vi "Main.vi"() -> ()   [LabVIEW 2018]
doc: "The myRIO Project template acquires acceleration data from the onboard accelerometer and displays the changes of acceleration values in a waveform chart."
uses:
  <vilib>/Platform/TimedLoop/XDataNode/timing_clust.ctl
  <vilib>/Platform/TimedLoop/XDataNode/nitl_modes.ctl
  <vilib>/Platform/TimedLoop/XDataNode/wakeup.ctl
  <vilib>/myRIO/Instrument Drivers/Onboard IO/DIO/typedefs/DIO Reference.ctl
  <vilib>/myRIO/Common/Instrument Driver Framework/Utilities/typedefs/myRIO Generic Hardware Reference.ctl
  <vilib>/myRIO/Common/Instrument Driver Framework/Utilities/typedefs/Hardware Version Enum.ctl
  <vilib>/myRIO/Common/Instrument Driver Framework/Utilities/typedefs/myRIO v1.0 Reference.ctl
  <vilib>/myRIO/Common/Instrument Driver Framework/Utilities/typedefs/Generic FPGA Reference.ctl
  <vilib>/myRIO/Common/Instrument Driver Framework/myRIO v1.0/DIO/typedefs/DIO Channels List.ctl
  <vilib>/myRIO/Common/Instrument Driver Framework/myRIO v1.0/DIO/typedefs/DIO Channels Enum.ctl
  <vilib>/userdefined/High Color/nirio_resource_hc.ctl
  <vilib>/myRIO/Instrument Drivers/Onboard IO/AI/typedefs/AI Reference.ctl
  <vilib>/myRIO/Common/Instrument Driver Framework/myRIO v1.0/AI/typedefs/AI Channels List.ctl
  <vilib>/myRIO/Common/Instrument Driver Framework/myRIO v1.0/AI/typedefs/AI Channels Enum.ctl
  <vilib>/myRIO/Common/Instrument Driver Framework/Utilities/typedefs/Analog Scaling Constants List.ctl
  <vilib>/myRIO/Common/Instrument Driver Framework/Utilities/typedefs/Analog Scaling Constants.ctl
  <vilib>/myRIO/Instrument Drivers/Onboard IO/AO/typedefs/AO Reference.ctl
  <vilib>/myRIO/Common/Instrument Driver Framework/myRIO v1.0/AO/typedefs/AO Channels List.ctl
  <vilib>/myRIO/Common/Instrument Driver Framework/myRIO v1.0/AO/typedefs/AO Channels Enum.ctl
  <vilib>/myRIO/Common/Instrument Driver Framework/Utilities/vis/Is FPGA Ref Available.vi
  <vilib>/myRIO/Common/Instrument Driver Framework/myRIO v1.0/AI/vis/myRIO v1.1 Open AI.vi
  <vilib>/myRIO/Instrument Drivers/Onboard IO/AI/vis/Read.vi
  <vilib>/myRIO/Common/Instrument Driver Framework/myRIO v1.0/AO/vis/myRIO v1.1 Open AO.vi
  <vilib>/myRIO/Instrument Drivers/Onboard IO/AO/vis/Write.vi
  <vilib>/myRIO/Common/Instrument Driver Framework/myRIO v1.0/DIO/vis/myRIO v1.1 Open DIO.vi
  <vilib>/myRIO/Instrument Drivers/Onboard IO/DIO/vis/Write.vi
  <vilib>/myRIO/Instrument Drivers/Onboard IO/DIO/vis/Read.vi
  <vilib>/myRIO/Common/Instrument Driver Framework/Utilities/vis/Validate Channels.vi
  <vilib>/myRIO/Common/Instrument Driver Framework/myRIO v1.0/AI/vis/myRIO v1.0 Reserve AI.vi
  <vilib>/myRIO/Common/Instrument Driver Framework/myRIO v1.0/AO/vis/myRIO v1.0 Reserve AO.vi
  <vilib>/myRIO/Common/Instrument Driver Framework/myRIO v1.0/DIO/vis/myRIO v1.0 Reserve DIO.vi
  <vilib>/myRIO/Common/Instrument Driver Framework/myRIO v1.0/AI/vis/myRIO v1.0 Build MUX Configuration AI.vi
  <vilib>/myRIO/Common/Instrument Driver Framework/myRIO v1.0/Resource Manager/vis/myRIO v1.0 Reserve Channel List.vi
  <vilib>/myRIO/Common/Instrument Driver Framework/myRIO v1.0/AO/vis/myRIO v1.0 Build MUX Configuration AO.vi
  <vilib>/myRIO/Common/Instrument Driver Framework/myRIO v1.0/DIO/vis/myRIO v1.0 Build MUX Configuration DIO.vi
  <vilib>/myRIO/Common/Instrument Driver Framework/myRIO v1.0/Resource Manager/vis/myRIO v1.0 Reserve Channel.vi
  <vilib>/myRIO/Common/Instrument Driver Framework/myRIO v1.0/Resource Manager/vis/myRIO v1.0 Unreserve Channel.vi
  <vilib>/myRIO/Common/Instrument Driver Framework/myRIO v1.0/Resource Manager/vis/myRIO v1.0 Create Configuration List.vi
  <vilib>/myRIO/Common/Instrument Driver Framework/myRIO v1.0/Resource Manager/vis/myRIO v1.0 Build Mutex Name.vi
  <vilib>/functionblocks/Counter/Pulse Timer/Pulse Timer.vi
  <vilib>/Utility/VariantDataType/GetNumericInfo.vi
  <vilib>/Utility/error.llb/Error Cluster From Error Code.vi
  <vilib>/myRIO/Common/Instrument Driver Framework/myRIO v1.0/myRIO v1.1 Open.vi
  <vilib>/myRIO/Common/Instrument Driver Framework/myRIO v1.0/AI/vis/myRIO v1.0 Get Scaling Constants AI.vi
  <vilib>/myRIO/Common/Instrument Driver Framework/Utilities/vis/IO Manager.vi
  <vilib>/myRIO/Common/Instrument Driver Framework/Utilities/vis/Configuration Manager.vi
  <vilib>/myRIO/Common/Instrument Driver Framework/myRIO v1.0/myRIO v1.0 Close.vi
  <vilib>/myRIO/Common/Instrument Driver Framework/myRIO v1.0/AI/vis/myRIO v1.0 Read AI.vi
  <vilib>/myRIO/Common/Instrument Driver Framework/myRIO v1.0/Resource Manager/vis/myRIO v1.0 Configure IO.vi
  <vilib>/myRIO/Common/Instrument Driver Framework/myRIO v1.0/DIO/vis/myRIO v1.0 Write DIO.vi
  <vilib>/myRIO/Common/Instrument Driver Framework/myRIO v1.0/DIO/vis/myRIO v1.0 Read DIO.vi
  <vilib>/functionblocks/Bistables/SR Bistable/SR Bistable.vi
  <vilib>/myRIO/Common/Instrument Driver Framework/myRIO v1.0/AO/vis/myRIO v1.0 Get Scaling Constants AO.vi
  <vilib>/myRIO/Common/Instrument Driver Framework/myRIO v1.0/AO/vis/myRIO v1.0 Write AO.vi
  <vilib>/Utility/file.llb/Write Delimited Spreadsheet (string).vi
  <vilib>/Platform/TimedLoop/XDataNode/XDataNode.xnode
  <vilib>/functionblocks/FB Core/FB Core.xnode
  <vilib>/myRIO/Express VI/Onboard IO/AI/AI Express VI.xnode
  <vilib>/myRIO/Instrument Drivers/Onboard IO/AI/vis/myRIO AI Open.xnode
  <vilib>/myRIO/Express VI/Onboard IO/DO/DO Express VI.xnode
  <vilib>/myRIO/Instrument Drivers/Onboard IO/DIO/vis/myRIO DIO Open.xnode
  <vilib>/myRIO/Express VI/Onboard IO/DI/DI Express VI.xnode
  <vilib>/myRIO/Express VI/Onboard IO/AO/AO Express VI.xnode
  <vilib>/myRIO/Instrument Drivers/Onboard IO/AO/vis/myRIO AO Open.xnode
  <vilib>/myRIO/Express VI/Onboard Devices/LED/LED Express VI.xnode
  <vilib>/myRIO/Instrument Drivers/Onboard IO/DIO/DIO.lvlib
  <vilib>/myRIO/Instrument Drivers/Onboard IO/AI/AI.lvlib
  <vilib>/myRIO/Instrument Drivers/Onboard IO/AO/AO.lvlib
  <vilib>/functionblocks/NI_FunctionBlock Libraries.lvlib
  <vilib>/Platform/TimedLoop/XDataNode/XDNodeRunTimeDep.lvlib
panel:
  out "AOUT":dbl
  out "AIN":dbl
  in  "Pump Test":bool
  out "APPS fault":bool
  out "APPS Output (V)":dbl
  out "APPS output %":dbl
  out "Accelaration":dbl(knob) scale=0.0..100.0
  out "APPS pedal travel %":dbl
  out "APPS2 (V) Input (B/AI1 (Pin 5)) 2":dbl
  out "APPS1":dbl(knob) scale=0.0..100.0
  out "APPS2":dbl(knob) scale=0.0..100.0
  out "APPS2 % 2":dbl
  out "APPS1 (V) Input (B/AI1 (Pin 5)) 2":dbl
  out "APPS1 % 2":dbl
  out "Pump out":bool
  out "RTD Status LED":bool
  out "RFE Indicator":bool
  out "AIR + Boolean":bool
  out "AIR +(A9)":dbl
  out "RTD Button":bool
  out "RTD Brake":bool
  out "EN Indicator":bool
  out "RTD Buzzer":bool
  in  "Buzzer test":bool
  in  "RTD Brake Test":bool
  in  "RFE  Test":bool
  in  "EN Test":bool
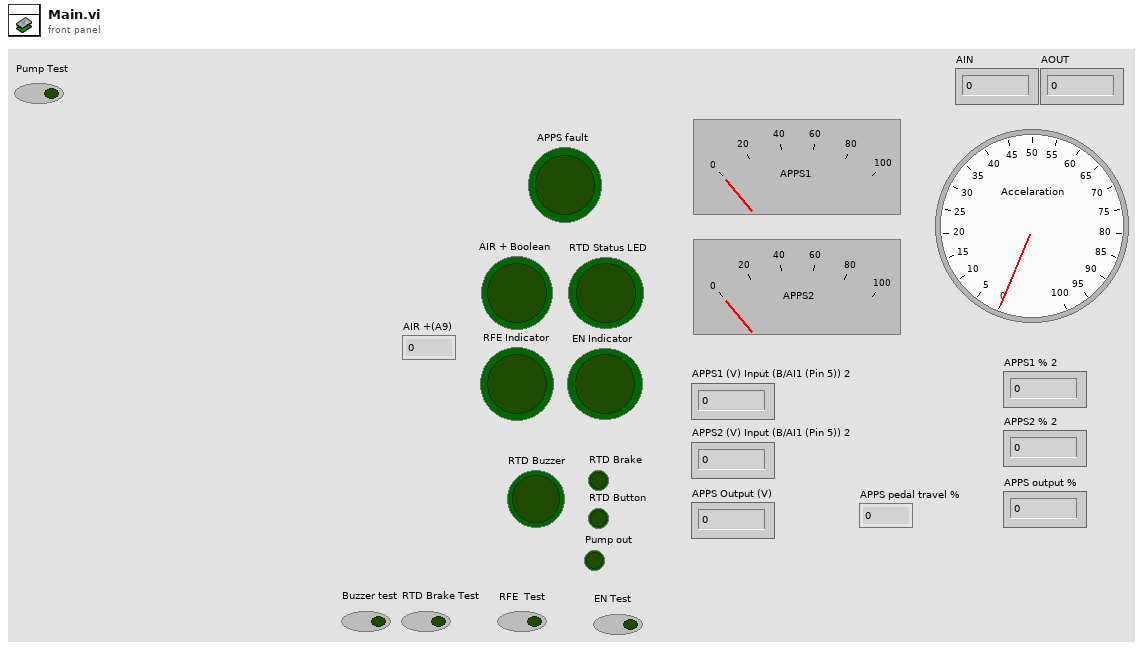
[diagram p1: front panel]
types:
  T1 = typedef "XDNodeRunTimeDep.lvlib/timing_clust.ctl" = cluster{"Expected End [f-1]":u64, "Actual End [f-1]":u64, "Finished Late? [f-1]":bool, "Expected End [i-1]":u64, "Actual End [i-1]":u64, "Finished Late? [i-1]":bool, "Expected Start [i]":u64, "Actual Start [i]":u64, "Expected Start [f]":u64, "Actual Start [f]":u64, "Source Name":string, "Structure Name":string, "Period":i64, "Deadline":i64, "Offset":i64, "Start":i64, "Priority":i32, "Timeout":i32, "Mode":T2, "Wakeup Reason":T3, "Error":errorcluster, "Source Type":string, "Secondary Source Type":string, "Global End Time":u64, "Global Start Time":u64, "Frame Duration":u64, "Iteration Duration":u64, "Assigned CPU":i32, "I/O Scan Engine Mode":u32}
  T2 = typedef "XDNodeRunTimeDep.lvlib/nitl_modes.ctl" = enum32{"No Change", "Process missed periods, maintain original phase", "Discard missed periods, maintain original phase", "Process missed periods, ignore original phase", "Discard missed periods, ignore original phase"}
  T3 = typedef "XDNodeRunTimeDep.lvlib/wakeup.ctl" = enum32{"Normal", "Aborted", "Asynchronous wakeup", "Timing source error", "Timed loop error", "Timeout"}
  T4 = typedef "AO.lvlib/AO Reference.ctl" = cluster{"myRIO Reference":T5, "AO Channel List":T9, "AO Scaling Constant List":T11}
  T5 = typedef "myRIO Generic Hardware Reference.ctl" = cluster{"myRIO Model":T6, "myRIO Hardware Reference":T7}
  T6 = typedef "Hardware Version Enum.ctl" = enum16{"Unknown", "myRIO-1900", "myRIO-1950", "roboRIO", "NI ELVIS RIO CM", "ELVIS III"}
  T7 = typedef "myRIO v1.0 Reference.ctl" = cluster{"Generic FPGA Reference":T8, "Allow multiple opens":bool}
  T8 = typedef "Generic FPGA Reference.ctl" = refnum<k20>
  T9 = typedef "AO Channels List.ctl" = T10[]
  T10 = typedef "AO Channels Enum.ctl" = enum16{"Not Connected", "AudioOut/Left", "AudioOut/Right", "C/AO0", "C/AO1", "A/AO0", "A/AO1", "B/AO0", "B/AO1"}
  T11 = typedef "Analog Scaling Constants List.ctl" = T12[]
  T12 = typedef "Analog Scaling Constants.ctl" = cluster{"LSB Weight (Volts)":dbl, "Offset (Volts)":dbl, "Signed?":bool}
  T13 = typedef "nirio_resource_hc.ctl" = tag
  T14 = typedef "AI.lvlib/AI Reference.ctl" = cluster{"myRIO Reference":T5, "AI Channels List":T15, "AI Scaling Constants List":T11}
  T15 = typedef "AI Channels List.ctl" = T16[]
  T16 = typedef "AI Channels Enum.ctl" = enum16{"Not Connected", "AudioIn/Left", "AudioIn/Right", "C/AI0", "C/AI1", "A/AI0", "A/AI1", "A/AI2", "A/AI3", "A/AI4", "A/AI5", "A/AI6", "A/AI7", "B/AI0", "B/AI1", "B/AI2", "B/AI3", "B/AI4", "B/AI5", "B/AI6", "B/AI7", "AI/AI0", "AI/AI1", "AI/AI2", "AI/AI3", "A/AI0 (DIFF)", "A/AI1 (DIFF)", "A/AI2 (DIFF)", "A/AI3 (DIFF)", "B/AI0 (DIFF)", "B/AI1 (DIFF)", "B/AI2 (DIFF)", "B/AI3 (DIFF)"}
  T17 = typedef "DIO.lvlib/DIO Reference.ctl" = cluster{"myRIO Reference":T5, "DIO Channels List":T18}
  T18 = typedef "DIO Channels List.ctl" = T19[]
  T19 = typedef "DIO Channels Enum.ctl" = enum16{"Not Connected", "C/DIO0", "C/DIO1", "C/DIO2", "C/DIO3", "C/DIO4", "C/DIO5", "C/DIO6", "C/DIO7", "A/DIO0", "A/DIO1", "A/DIO2", "A/DIO3", "A/DIO4", "A/DIO5", "A/DIO6", "A/DIO7", "A/DIO8", "A/DIO9", "A/DIO10", "A/DIO11", "A/DIO12", "A/DIO13", "A/DIO14", "A/DIO15", "A/DIO16", "A/DIO17", "A/DIO18", "A/DIO19", "B/DIO0", "B/DIO1", "B/DIO2", "B/DIO3", "B/DIO4", "B/DIO5", "B/DIO6", "B/DIO7", "B/DIO8", "B/DIO9", "B/DIO10", "B/DIO11", "B/DIO12", "B/DIO13", "B/DIO14", "B/DIO15", "B/DIO16", "B/DIO17", "B/DIO18", "B/DIO19", "LED0", "LED1", "LED2", "LED3", "Button0", "DIO/DIO0", "DIO/DIO1", "DIO/DIO2", "DIO/DIO3", "DIO/DIO4", "DIO/DIO5", "DIO/DIO6", "DIO/DIO7", "DIO/DIO8", "DIO/DIO9", "SPI/CS0", "SPI/CS1", "SPI/CS2", "SPI/CS3", "LED RADIO (Green)", "LED RADIO (Red)", "LED COMM (Green)", "LED COMM (Red)", "LED MODE (Green)", "LED MODE (Red)"}
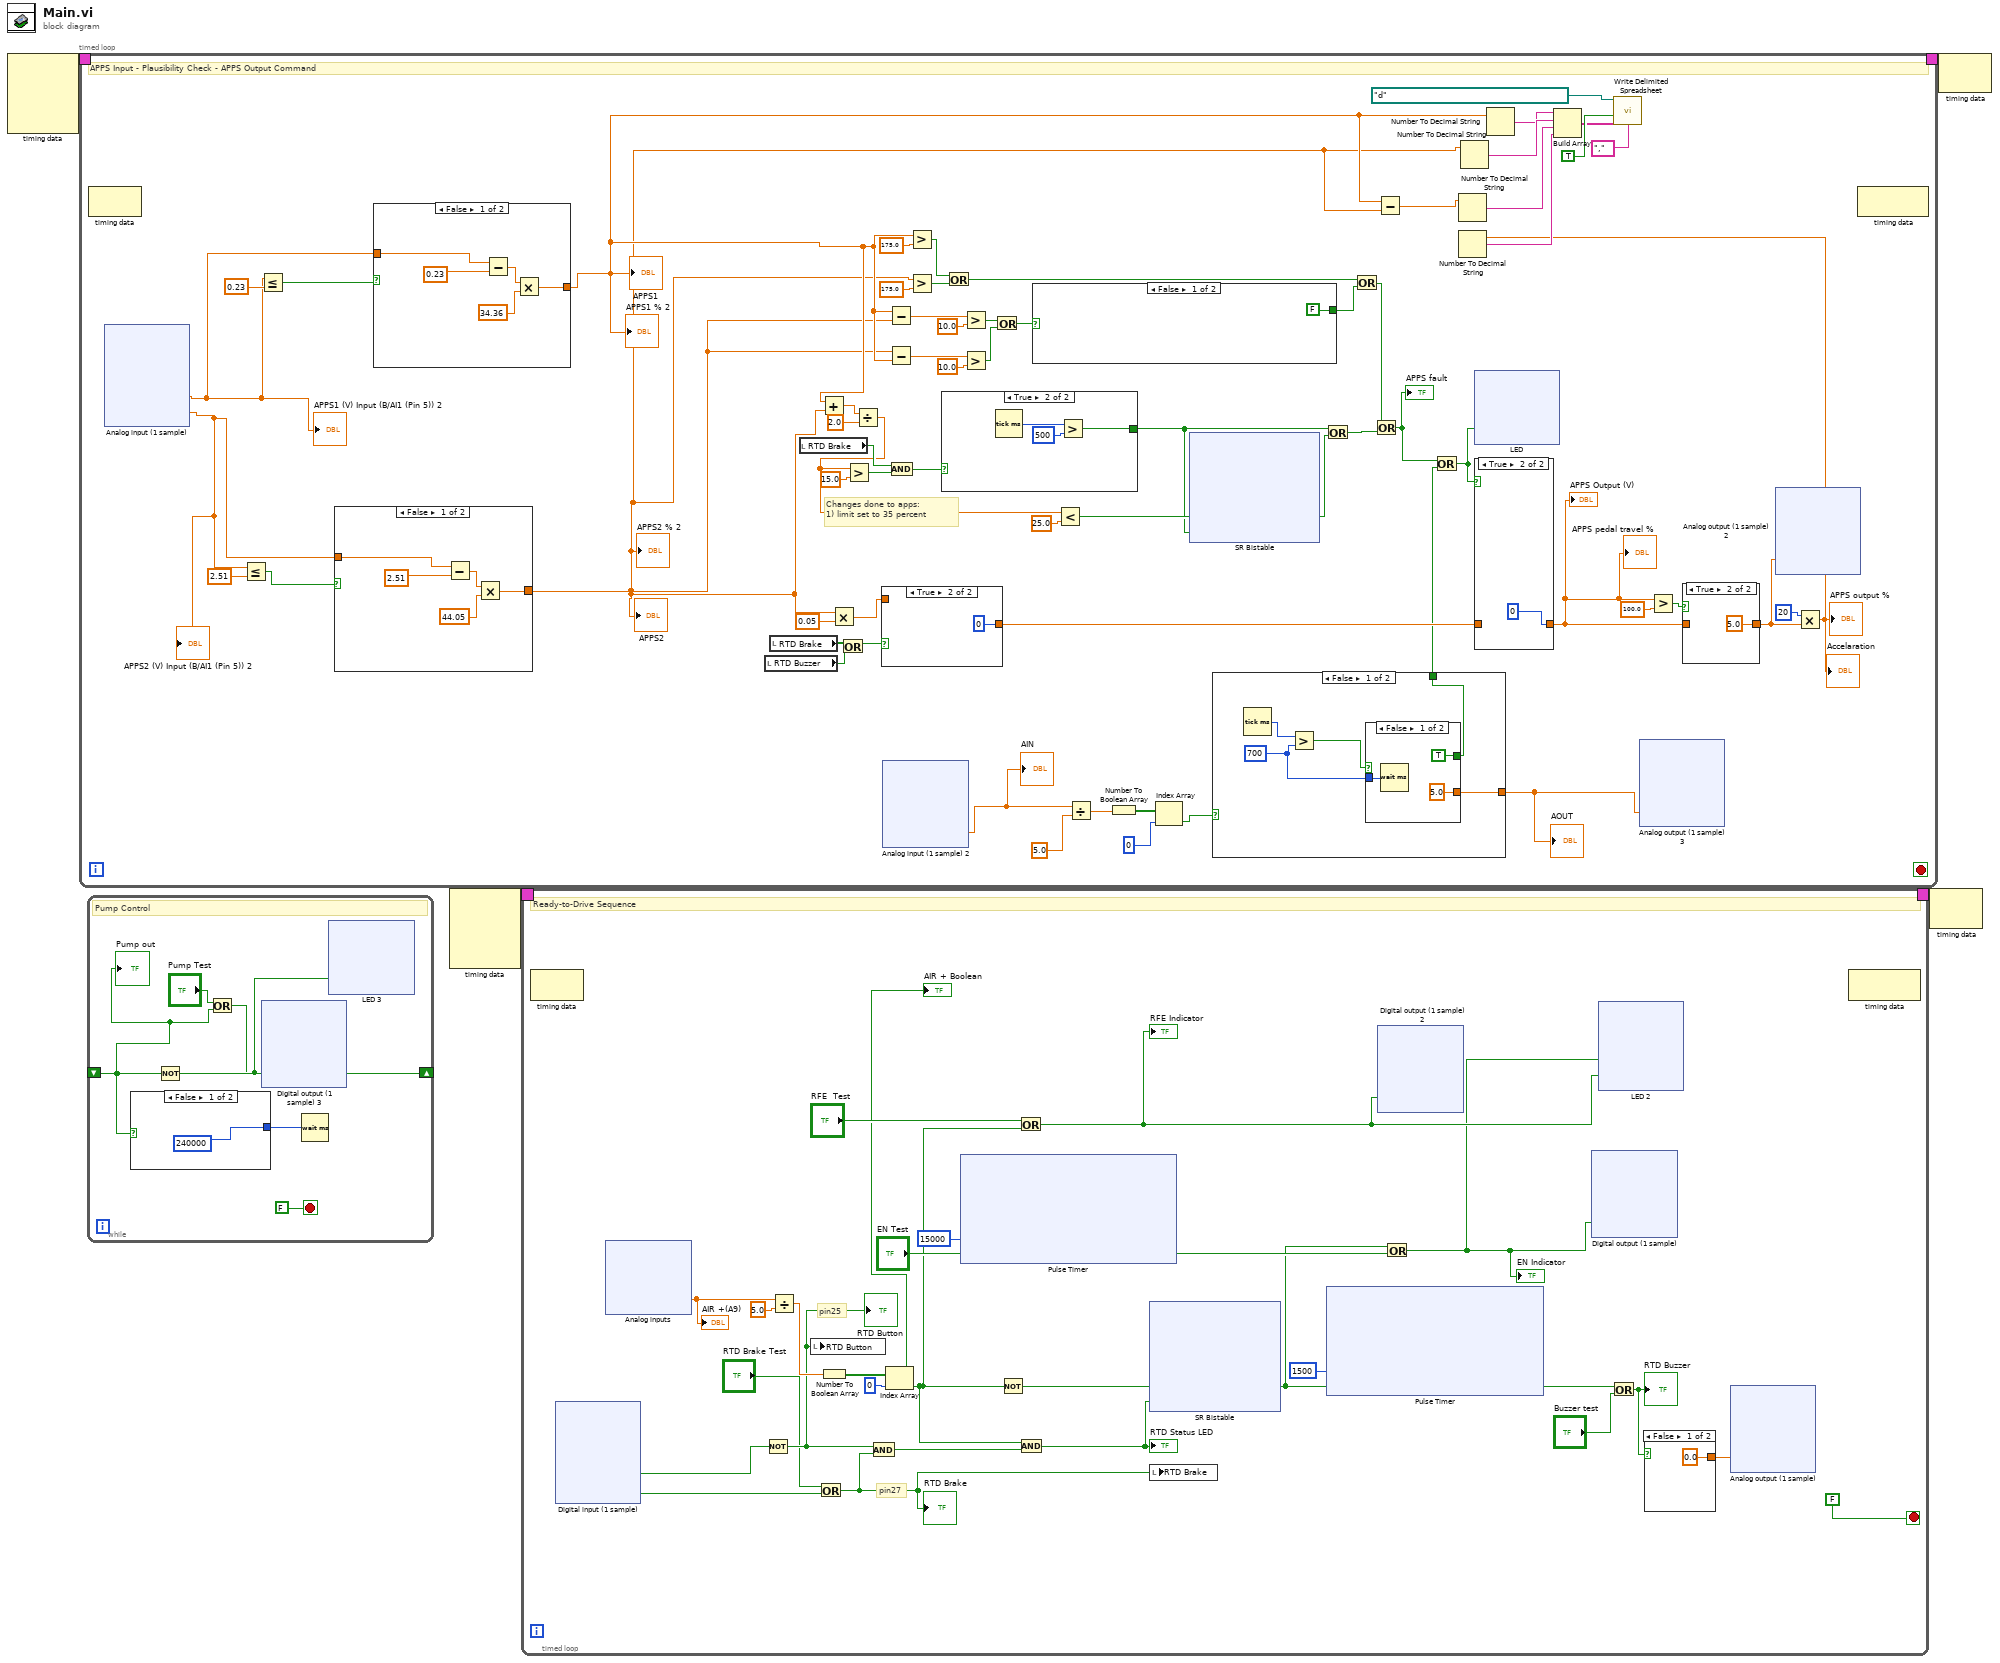
[diagram p0: block diagram]
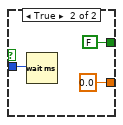
[diagram p2: hidden frame]
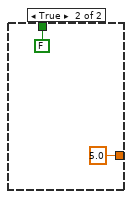
[diagram p3: hidden frame]
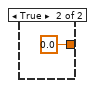
[diagram p4: hidden frame]
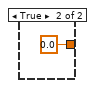
[diagram p5: hidden frame]
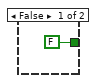
[diagram p6: hidden frame]
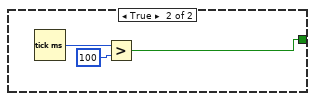
[diagram p7: hidden frame]
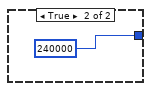
[diagram p11: hidden frame]
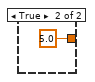
[diagram p12: hidden frame]
diagram:
  n1 = node-c288() -> (w2:T1)  [unwired: 4 in]
  n2 = timed-loop {
    timing: w2 -> [_]
    timing-out: [_] -> w1
    stop <- _ stop-if-true
    # "Changes done to apps:\n1) limit set to 35 percent"
    # "APPS Input - Plausibility Check - APPS Output Command"
    n3 = node-c288() -> ()  [unwired: 1 in, 1 out]
    n4 = xnode "Analog input (1 sample)"() -> ("APPS 1 Input (A/AI2 (Pin 7))"=w16:dbl, "APPS 2 Input (A/AI1 (Pin 5))"=w15:dbl)  [unwired: 1 in, 1 out]
    "APPS2 (V) Input (B/AI1 (Pin 5)) 2" <- w15
    "APPS1 (V) Input (B/AI1 (Pin 5)) 2" <- w16
    n5 = Less Or Equal?(x=w15, y=2.51) -> (x <= y?=w35:bool)
    n6 = Less Or Equal?(x=w16, y=0.23) -> (x <= y?=w33:bool)
    n7 = case shown="False" w35 {
      tunnel: w15 -> [w163 _]
      tunnel: [w162 0.0] -> w21
      frame False {
        n8 = Subtract(x=w163, y=2.51) -> (x-y=w165:dbl)
        n9 = Multiply(x=w165, y=44.05) -> (x*y=w162:dbl)
      }
      frame True {
      }
    }
    "APPS2" <- w21
    "APPS2 % 2" <- w21
    n10 = case shown="False" w33 {
      tunnel: w16 -> [w157 _]
      tunnel: [w156 0.0] -> w22
      frame False {
        n11 = Subtract(x=w157, y=0.23) -> (x-y=w159:dbl)
        n12 = Multiply(x=w159, y=34.36) -> (x*y=w156:dbl)
      }
      frame True {
      }
    }
    "APPS1" <- w22
    "APPS1 % 2" <- w22
    n13 = local read "RTD Buzzer"() -> (w38:bool)
    n14 = local read "RTD Brake"() -> (w32:bool)
    n15 = local read "RTD Brake"() -> (w46:bool)
    n16 = Add(x=w22, y=w21) -> (x+y=w41:dbl)
    n17 = Multiply(x=w21, y=0.05) -> (x*y=w29:dbl)
    n18 = Or(x=w32, y=w38) -> ()  [unwired: 1 out]
    n19 = Divide(x=w41, y=2.0) -> (x/y=w39:dbl)
    n20 = Greater?(x=w39, y=15.0) -> (0:w56:bool)
    n21 = case shown="True" w32 {
      tunnel: [w258 0] -> w53
      tunnel: w29 -> [w258 _]
      frame False {
      }
      frame True {
      }
    }
    n22 = xnode "Analog input (1 sample) 2"() -> ("AI (A/AI0 (Pin 3))"=w14:dbl)  [unwired: 1 in, 1 out]
    "AIN" <- w14
    n23 = Subtract(x=w22, y=w21) -> (x-y=w66:dbl)
    n24 = Subtract(x=w21, y=w22) -> (x-y=w58:dbl)
    n25 = And(x=w46, y=w56) -> (x .and. y?=w43:bool)
    n26 = Greater?(x=w22, y=175.0) -> (0:w63:bool)
    n27 = Greater?(x=w21, y=175.0) -> (0:w62:bool)
    n28 = case shown="True" w43 {
      tunnel: [FALSE w209] -> w42
      frame False {
      }
      frame True {
        n29 = Tick Count (ms)() -> (millisecond timer value=w211:u32)
        n30 = Greater?(x=w211, y=u32 500) -> (0:w209:bool)
      }
    }
    n31 = Or(x=w63, y=w62) -> (x .or. y?=w61:bool)
    n32 = Greater?(x=w66, y=10.0) -> (0:w67:bool)
    n33 = Greater?(x=w58, y=10.0) -> (0:w59:bool)
    n34 = Or(x=w67, y=w59) -> (x .or. y?=w50:bool)
    n35 = case shown="False" w50 {
      tunnel: [FALSE w255] -> w49
      frame False {
      }
      frame True {
        n36 = Tick Count (ms)() -> (millisecond timer value=w257:u32)
        n37 = Greater?(x=w257, y=u32 100) -> (0:w255:bool)
      }
    }
    n38 = Less?(x=w39, y=25.0) -> (x < y?=w47:bool)
    n39 = Divide(x=w14, y=5.0) -> (x/y=w12:dbl)
    n40 = Number To Boolean Array(number=w12) -> (Boolean array=w11:bool[])
    n41 = Index Array(array=w11, index=0) -> (element=w9:bool)
    n42 = xnode "SR Bistable"("reset"=w47, "set"=w42) -> ("output"=w48:bool)  [unwired: 1 in, 1 out]
    n43 = case shown="False" w9 {
      tunnel: [w108 5.0] -> w5
      tunnel: [w107 FALSE] -> w8
      frame False {
        w106 = u32 700 ("y")
        n44 = Tick Count (ms)() -> (millisecond timer value=w109:u32)
        n45 = Greater?(x=w109, y=w106) -> (0:w110:bool)
        n46 = case shown="False" w110 {
          tunnel: [5.0 0.0] -> w108
          tunnel: [TRUE FALSE] -> w107
          tunnel: w106 -> [w111 w114]
          frame False {
            n47 = Wait (ms)(milliseconds to wait=w111) -> ()  [unwired: 1 out]
          }
          frame True {
            n48 = Wait (ms)(milliseconds to wait=w114) -> ()  [unwired: 1 out]
          }
        }
      }
      frame True {
      }
    }
    "AOUT" <- w5
    n49 = Or(x=w42, y=w48) -> (x .or. y?=w44:bool)
    n50 = Or(x=w61, y=w49) -> (x .or. y?=w45:bool)
    n51 = Or(x=w45, y=w44) -> (x .or. y?=w7:bool)
    "APPS fault" <- w7
    n52 = Subtract(x=w22, y=w21) -> (x-y=w20:dbl)
    n53 = Or(x=w7, y=w8) -> (x .or. y?=w6:bool)
    n54 = Number To Decimal String(number=w20) -> (decimal integer string=w23:string)  [unwired: 1 in]
    n55 = Number To Decimal String(number=w21) -> (decimal integer string=w28:string)  [unwired: 1 in]
    n56 = xnode "LED"("LED0"=w6) -> ()  [unwired: 1 in, 1 out]
    n57 = case shown="True" w6 {
      tunnel: w53 -> [w262 _]
      tunnel: [w262 0] -> w31
      frame False {
      }
      frame True {
      }
    }
    "APPS Output (V)" <- w31
    "APPS pedal travel %" <- w31
    n58 = Number To Decimal String(number=w22) -> (decimal integer string=w27:string)  [unwired: 1 in]
    n59 = xnode "Analog output (1 sample) 3"("A/AO0 (Pin 2)"=w5) -> ()  [unwired: 1 in, 1 out]
    n60 = Greater?(x=w31, y=100.0) -> (0:w54:bool)
    n61 = case shown="True" w54 {
      tunnel: [w260 5.0 ("APPS output %")] -> w37
      tunnel: w31 -> [w260 _]
      frame False {
      }
      frame True {
      }
    }
    n62 = xnode "Analog output (1 sample) 2"("APPS Output (B/AO0 (Pin 2))"=w37) -> ()  [unwired: 1 in, 1 out]
    n63 = Multiply(x=20, y=w37) -> (x*y=w18:dbl)
    "APPS output %" <- w18
    "Accelaration" <- w18
    n64 = Number To Decimal String(number=w18) -> (decimal integer string=w19:string)  [unwired: 1 in]
    n65 = Build Array(w27, w28, w23, w19) -> (w17:string[])
    n66 = call-poly <vilib>:"Write Delimited Spreadsheet.vi"("file path (dialog if empty)"=path "d:/", "1D data"=w17, "append to file? (new file:F)"=TRUE, "delimiter (\\t)"="," ("delimiter (\\t)")) -> ()  [unwired: 10 in, 2 out]
    n67 = node-c288() -> ()  [unwired: 1 in, 1 out]
  }
  n68 = while {
    shift-right: [w341] -> _
    shift-left: _ -> [w337]
    stop <- FALSE stop-if-true
    # "Pump Control"
    n69 = case shown="False" w337 {
      tunnel: [240000 240000] -> w340
      frame False {
      }
      frame True {
      }
    }
    n70 = Not(x=w337) -> (.not. x?=w341:bool)
    n71 = Or(x="Pump Test", y=w337) -> (x .or. y?=w336:bool)
    n72 = xnode "Digital output (1 sample) 3"("Pump out (B/DIO7 (Pin 25))"=w336) -> ()  [unwired: 1 in, 1 out]
    n73 = Wait (ms)(milliseconds to wait=w340) -> ()  [unwired: 1 out]
    n74 = xnode "LED 3"("PUMP"=w336) -> ()  [unwired: 1 in, 1 out]
    "Pump out" <- w337
  }
  n75 = node-c288() -> (w4:T1)  [unwired: 4 in]
  n76 = timed-loop {
    timing: w4 -> [_]
    timing-out: [_] -> w3
    stop <- FALSE stop-if-true
    # "pin27"
    # "pin25"
    # "Ready-to-Drive Sequence"
    n77 = node-c288() -> ()  [unwired: 1 in, 1 out]
    n78 = xnode "Digital input (1 sample)"() -> ("RTD Button (B/DIO2 (Pin 15))"=w435:bool, "RTD Brake (B/DIO3 (Pin 17))"=w416:bool)  [unwired: 1 in, 1 out]
    n79 = xnode "Analog inputs"() -> ("AIR + (A/AI3 (Pin 9))"=w419:dbl)  [unwired: 1 in, 1 out]
    "AIR +(A9)" <- w419
    n80 = Not(x=w435) -> (.not. x?=w433:bool)
    "RTD Button" <- w433
    n81 = Divide(x=w419, y=5.0) -> (x/y=w439:dbl)
    n82 = local write "RTD Button"(w433) -> ()
    n83 = Or(x="RTD Brake Test", y=w416) -> (x .or. y?=w430:bool)
    "RTD Brake" <- w430
    n84 = Number To Boolean Array(number=w439) -> (Boolean array=w440:bool[])
    n85 = And(x=w433, y=w430) -> (x .and. y?=w436:bool)
    n86 = Index Array(array=w440, index=0) -> (element=w415:bool)
    "AIR + Boolean" <- w415
    n87 = xnode "Pulse Timer"("preset time (ms)"=15000, "input"="EN Test") -> ("output"=w427:bool)  [unwired: 1 in, 2 out]
    n88 = Not(x=w415) -> (.not. x?=w414:bool)
    n89 = Or(x="RFE  Test", y=w415) -> (x .or. y?=w418:bool)
    "RFE Indicator" <- w418
    n90 = And(x=w415, y=w436) -> (x .and. y?=w432:bool)
    "RTD Status LED" <- w432
    n91 = xnode "SR Bistable"("reset"=w414, "set"=w432) -> ("output"=w425:bool)  [unwired: 1 in, 1 out]
    n92 = local write "RTD Brake"(w430) -> ()
    n93 = xnode "Pulse Timer"("preset time (ms)"=1500, "input"=w425) -> ("output"=w423:bool)  [unwired: 1 in, 2 out]
    n94 = xnode "Digital output (1 sample) 2"("RFE (B/DIO0 (Pin 11))"=w418) -> ()  [unwired: 1 in, 1 out]
    n95 = Or(x=w425, y=w427) -> (x .or. y?=w417:bool)
    "EN Indicator" <- w417
    n96 = xnode "Digital output (1 sample)"("EN (B/DIO1 (Pin 13))"=w417) -> ()  [unwired: 1 in, 1 out]
    n97 = xnode "LED 2"("EN"=w417, "RFE"=w418) -> ()  [unwired: 1 in, 1 out]
    n98 = Or(x=w423, y="Buzzer test") -> (x .or. y?=w422:bool)
    "RTD Buzzer" <- w422
    n99 = case shown="False" w422 {
      tunnel: [0.0 ("y") 5.0 ("y")] -> w434
      frame False {
      }
      frame True {
      }
    }
    n100 = xnode "Analog output (1 sample)"("RTD - Buzzer (B/AO1 (Pin 4))"=w434) -> ()  [unwired: 1 in, 1 out]
    n101 = node-c288() -> ()  [unwired: 1 in, 1 out]
  }
  n102 = node-c288(w3) -> ()  [unwired: 1 out]
  n103 = node-c288(w1) -> ()  [unwired: 1 out]
